vi "Auto Check Each Tube Posibly Modded for Prevent Trip.vi"(6 "error in (no error)":errorcluster, 8 "BoardHandle in":T1, 9 "Barcodes in":string[](array[string]), 10 "Tube #":i32) -> (0 "Current 4":dbl, 1 "Current 3":dbl, 2 "Current 2":dbl, 3 "Current 1":dbl, 4 "error out":errorcluster, 5 "BoardHandle out":T1)   [LabVIEW 2020]
uses:
  Program Files/National Instruments/LabVIEW 2018/instr.lib/CAEN PSM/CAEN PSM.lvlib
panel:
  out "Actual Voltage Level (V) 2":dbl format="%#_13g"
  # "OUTPUTS"
  # "INPUTS"
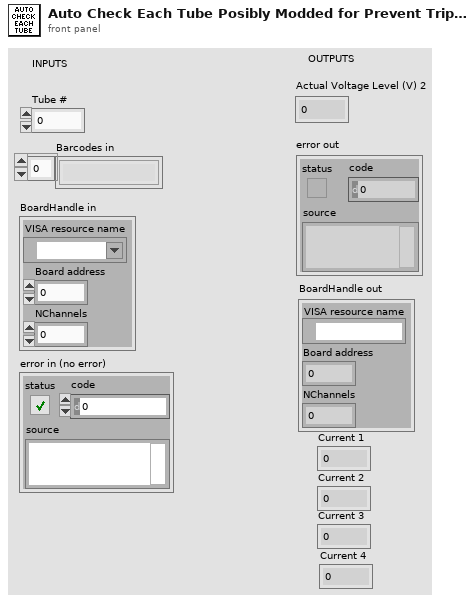
[diagram p1: front panel]
types:
  T1 = cluster{"VISA resource name":refnum<visa-resource-name>, "Board address":u8, "NChannels":u8}
  T2 = typedef "CAEN PSM.lvlib/BoardHandle.ctl" = cluster{"VISA resource name":refnum<visa-resource-name>, "Board address":u8, "NChannels":u8}
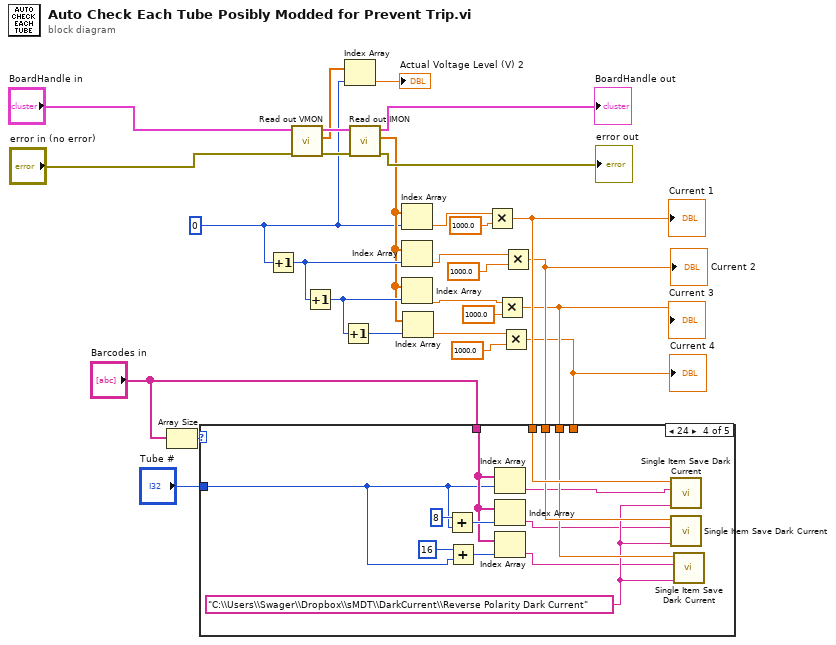
[diagram p0: block diagram]
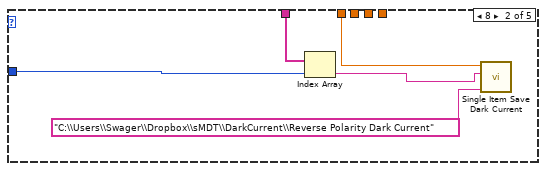
[diagram p3: hidden frame]
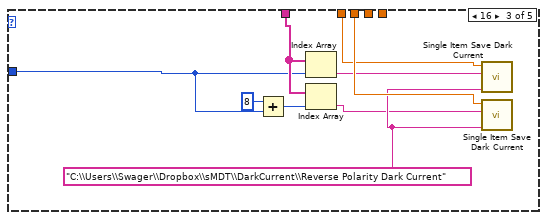
[diagram p4: hidden frame]
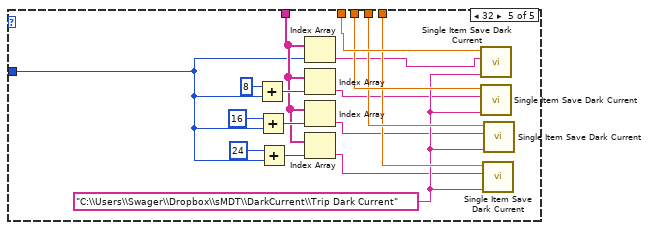
[diagram p5: hidden frame]
diagram:
  w14 = 0 ("index")
  n1 = Array Size(array="Barcodes in") -> (size(s)=w13:i32)
  n2 = Increment(x=w14) -> (x+1=w17:i32)
  n3 = call "Read out VMON.vi"("error in (no error)"="error in (no error)", "BoardHandle"="BoardHandle in") -> ("error out"=w25:errorcluster, "VMon values (V)"=w23:dbl[], "BoardHandle out"=w24:T2)  [unwired: 7 in]
  n4 = Increment(x=w17) -> (x+1=w16:i32)
  n5 = Increment(x=w16) -> (x+1=w18:i32)
  n6 = Index Array(array=w23, index=w14) -> (element=→"Actual Voltage Level (V) 2":dbl)
  n7 = call "Read out IMON.vi"("error in (no error)"=w25, "BoardHandle"=w24) -> ("error out"=→"error out":errorcluster, "IMon values (uA)"=w15:dbl[], "BoardHandle out"=→"BoardHandle out":T2)  [unwired: 6 in, 1 out]
  n8 = Index Array(array=w15, index=w14) -> (element=w26:dbl)
  n9 = Index Array(array=w15, index=w17) -> (element=w9:dbl)
  n10 = Index Array(array=w15, index=w16) -> (element=w5:dbl)
  n11 = Index Array(array=w15, index=w18) -> (element=w3:dbl)
  n12 = Multiply(x=w26, y=1000.0) -> (x*y=w12:dbl)
  "Current 1" <- w12
  n13 = Multiply(x=w5, y=1000.0) -> (x*y=w4:dbl)
  "Current 3" <- w4
  n14 = Multiply(x=w3, y=1000.0) -> (x*y=w1:dbl)
  "Current 4" <- w1
  n15 = Multiply(x=w9, y=1000.0) -> (x*y=w7:dbl)
  "Current 2" <- w7
  n16 = case shown="24" w13 {
    tunnel: w1 -> [_ _ _ _ w62]
    tunnel: w4 -> [_ _ _ w47 w63]
    tunnel: w7 -> [_ _ w38 w48 w64]
    tunnel: w12 -> [_ w31 w37 w49 w65]
    tunnel: "Barcodes in" -> [_ w33 w40 w51 w66]
    tunnel: "Tube #" -> [_ w32 w39 w50 w61]
    frame 0, Default {
    }
    frame 8 {
      n17 = Index Array(array=w33, index=w32) -> (element=w29:string)
      n18 = call "Single Item Save Dark Current.vi"("Filename"="C:\\Users\\Swager\\Dropbox\\sMDT\\DarkCurrent\\Reverse Polarity Dark Current", "Barcode"=w29, "Current"=w31) -> ()  [unwired: 9 in]
    }
    frame 16 {
      w36 = "C:\\Users\\Swager\\Dropbox\\sMDT\\DarkCurrent\\Reverse Polarity Dark Current" ("Filename")
      n19 = Add(x=8, y=w39) -> (x+y=w42:i32)
      n20 = Index Array(array=w40, index=w39) -> (element=w34:string)
      n21 = Index Array(array=w40, index=w42) -> (element=w35:string)
      n22 = call "Single Item Save Dark Current.vi"("Filename"=w36, "Barcode"=w34, "Current"=w37) -> ()  [unwired: 9 in]
      n23 = call "Single Item Save Dark Current.vi"("Filename"=w36, "Barcode"=w35, "Current"=w38) -> ()  [unwired: 9 in]
    }
    frame 24 {
      w46 = "C:\\Users\\Swager\\Dropbox\\sMDT\\DarkCurrent\\Reverse Polarity Dark Current" ("Filename")
      n24 = Add(x=8, y=w50) -> (x+y=w55:i32)
      n25 = Add(x=16, y=w50) -> (x+y=w53:i32)
      n26 = Index Array(array=w51, index=w50) -> (element=w43:string)
      n27 = Index Array(array=w51, index=w55) -> (element=w44:string)
      n28 = Index Array(array=w51, index=w53) -> (element=w45:string)
      n29 = call "Single Item Save Dark Current.vi"("Filename"=w46, "Barcode"=w43, "Current"=w49) -> ()  [unwired: 9 in]
      n30 = call "Single Item Save Dark Current.vi"("Filename"=w46, "Barcode"=w44, "Current"=w48) -> ()  [unwired: 9 in]
      n31 = call "Single Item Save Dark Current.vi"("Filename"=w46, "Barcode"=w45, "Current"=w47) -> ()  [unwired: 9 in]
    }
    frame 32 {
      w60 = "C:\\Users\\Swager\\Dropbox\\sMDT\\DarkCurrent\\Trip Dark Current" ("Filename")
      n32 = Add(x=8, y=w61) -> (x+y=w72:i32)
      n33 = Add(x=16, y=w61) -> (x+y=w70:i32)
      n34 = Add(x=24, y=w61) -> (x+y=w68:i32)
      n35 = Index Array(array=w66, index=w61) -> (element=w56:string)
      n36 = Index Array(array=w66, index=w72) -> (element=w57:string)
      n37 = Index Array(array=w66, index=w70) -> (element=w58:string)
      n38 = Index Array(array=w66, index=w68) -> (element=w59:string)
      n39 = call "Single Item Save Dark Current.vi"("Filename"=w60, "Barcode"=w56, "Current"=w65) -> ()  [unwired: 9 in]
      n40 = call "Single Item Save Dark Current.vi"("Filename"=w60, "Barcode"=w57, "Current"=w64) -> ()  [unwired: 9 in]
      n41 = call "Single Item Save Dark Current.vi"("Filename"=w60, "Barcode"=w59, "Current"=w62) -> ()  [unwired: 9 in]
      n42 = call "Single Item Save Dark Current.vi"("Filename"=w60, "Barcode"=w58, "Current"=w63) -> ()  [unwired: 9 in]
    }
  }
